vi "appendix_main.vi"() -> ()   [LabVIEW 2016]
uses:
  <vilib>/Utility/NIReport.llb/NI_report.lvclass
panel:
  out "error out":errorcluster
  in  "Reports folder":path=path "L:/Documentos/00 SERVIÇOS/Tensão residual/Olapa 10-2017/RelatóriosOlapa/Arquivos para o relatório"
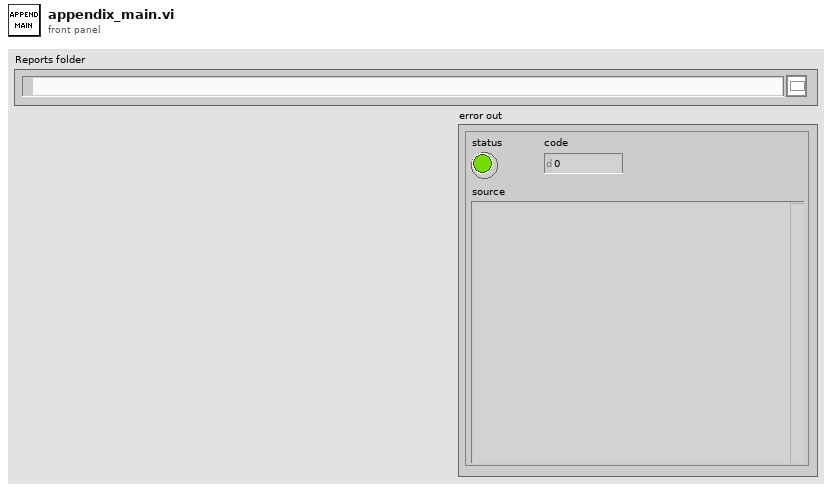
[diagram p1: front panel]
types:
  T1 = enum16{"Standard Report", "HTML", "Word", "Excel"}
  T2 = typedef "appendix_TableData.ctl" = cluster{"Title":string, "ColumHeaders":string[], "Data":string[][]}
  T3 = typedef "appendix_data.ctl" = cluster{"PathImage":path, "Legend":string, "tableData":T2}
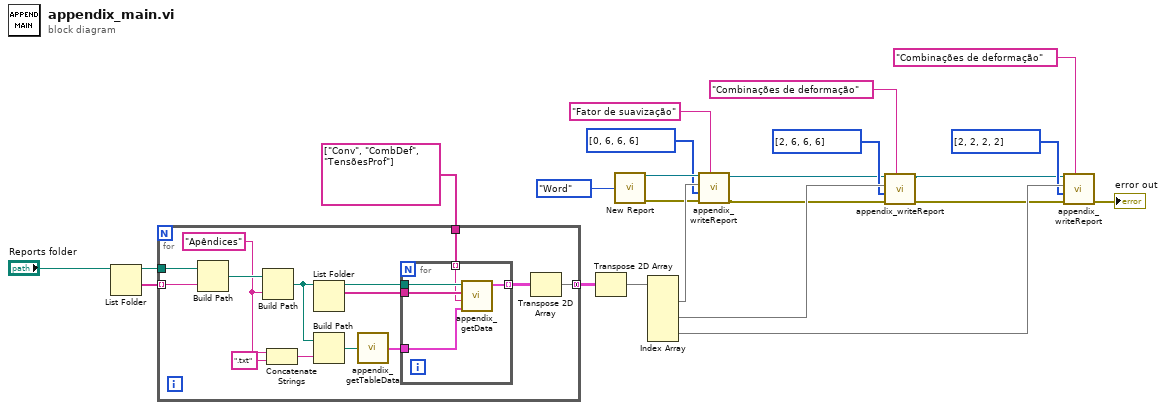
[diagram p0: block diagram]
diagram:
  n1 = List Folder(path="Reports folder") -> (path out=w21:path, folder names=w22:string[])  [unwired: 3 in, 2 out]
  n2 = for {
    tunnel: w22 -> [w37] mode=indexing
    tunnel: w21 -> [w36]
    tunnel: [w24] -> w20 mode=concatenating
    tunnel: string[] ["Conv", "CombDef", "TensõesProf"] ("Pattern") -> [w25]
    w30 = "Apêndices" ("name or relative path")
    n3 = Build Path(base path=w36, name or relative path=w37) -> (appended path=w35:path)
    n4 = Build Path(base path=w35, name or relative path=w30) -> (appended path=w32:path)
    n5 = Concatenate Strings(w30, ".txt" ("string")) -> (w31:string)
    n6 = List Folder(path=w32) -> (path out=w34:path, filenames=w33:string[])  [unwired: 3 in, 2 out]
    n7 = Build Path(base path=w32, name or relative path=w31) -> (appended path=w28:path)
    n8 = call "appendix_getTableData.vi"("appended path"=w28) -> ("TableData"=w27:T2[])
    n9 = for {
      tunnel: w34 -> [w42]
      tunnel: w33 -> [w41]
      tunnel: w27 -> [w40]
      tunnel: [w39] -> w26 mode=indexing
      tunnel: w25 -> [w38] mode=indexing
      n10 = call "appendix_getData.vi"("TableData"=w40, "Pattern"=w38, "filenames"=w41, "path in"=w42) -> ("Data"=w39:T3[])  [unwired: 7 in]
    }
    n11 = Transpose 2D Array(2D array=w26) -> (transposed array=w24:T3[][])
  }
  n12 = Transpose 2D Array(2D array=w20) -> (transposed array=w15:T3[][])
  n13 = call <vilib>:"New Report.vi"("report type"=T1."Word") -> ("report out"=w12:refnum<class "NI_report.lvclass">, "error out"=w13:errorcluster)  [unwired: 13 in]
  n14 = Index Array(array=w15) -> (element #1=w19:T3[], element #2=w17:T3[], element #3=w16:T3[])  [unwired: 6 in]
  n15 = call "appendix_writeReport.vi"("AppendixTitle"="Fator de suavização", "error in (no error)"=w13, "Precisions"=i16[] [0, 6, 6, 6], "Data"=w19, "NI_report in"=w12) -> ("error out"=w6:errorcluster, "Report out"=w7:refnum<class "NI_report.lvclass">)  [unwired: 5 in]
  n16 = call "appendix_writeReport.vi"("AppendixTitle"="Combinações de deformação", "error in (no error)"=w6, "Precisions"=i16[] [2, 6, 6, 6], "Data"=w17, "NI_report in"=w7) -> ("error out"=w3:errorcluster, "Report out"=w2:refnum<class "NI_report.lvclass">)  [unwired: 5 in]
  n17 = call "appendix_writeReport.vi"("AppendixTitle"="Combinações de deformação", "error in (no error)"=w3, "Precisions"=i16[] [2, 2, 2, 2], "Data"=w16, "NI_report in"=w2) -> ("error out"=→"error out":errorcluster)  [unwired: 5 in, 1 out]
